vi "Serial Port Close.vi"(8 "error in (no error)":errorcluster, 11 "Port handle":refnum<k24>) -> (0 "error out":errorcluster)   [LabVIEW 2015, in "VC940.lvlib"]
uses:
  VC940.lvlib
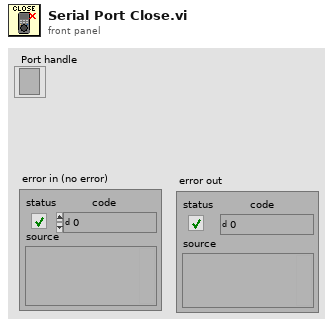
[diagram p1: front panel]
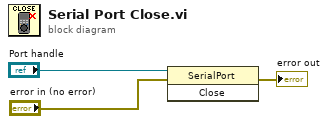
[diagram p0: block diagram]
diagram:
  n1 = invoke class="SerialPort" method="Close"(reference="Port handle", error in="error in (no error)") -> (error out=→"error out":errorcluster)  [unwired: 1 in, 2 out]
